vi "retrieveData.vi"(8 "error in (no error)":errorcluster, 11 "DistanceGauge in":refnum<class "DistanceGauge.lvclass">) -> (0 "error out":errorcluster, 2 "Distance Data":T1={"Distance Measured 1"=1.0, "Distance Measured 2"=1.0} {"Distance Measured 2" min=1.0 max=300.0 format="%.1f"; "Distance Measured 1" min=1.0 max=300.0 format="%.1f"}, 3 "DistanceGauge out":refnum<class "DistanceGauge.lvclass">)   [LabVIEW 2013, in "DistanceGauge.lvlib" / "DistanceGauge.lvclass"]
uses:
  <userlib>/Common/Devices/DistanceGauge/DistanceGauge/DistanceGauge.lvclass
  <userlib>/Common/Devices/DistanceGauge/Typedefs/Distance Data.ctl
  <userlib>/Common/Devices/DistanceGauge/DistanceGauge/DistanceGauge.lvclass/DistanceGauge.ctl
  <userlib>/Common/SerialProtocols/SerialCommunicator/SerialCommunicator.lvclass
  <userlib>/Common/Devices/DistanceGauge/DistanceGauge.lvlib
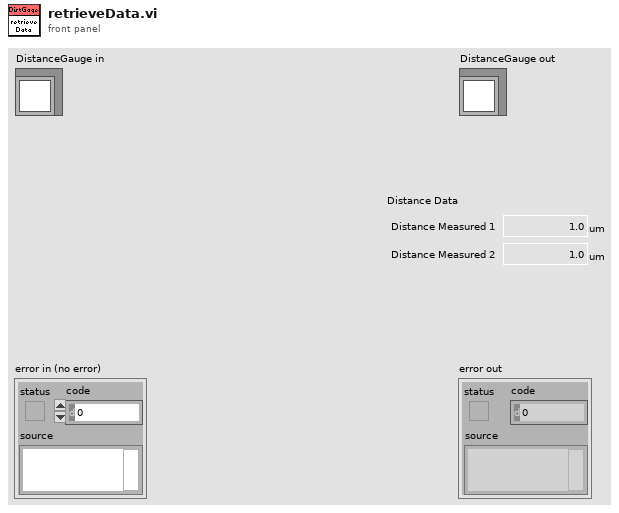
[diagram p1: front panel]
types:
  T1 = typedef "DistanceGauge.lvlib/Distance Data.ctl" = cluster{"Distance Measured 1":dbl[unit], "Distance Measured 2":dbl[unit]}
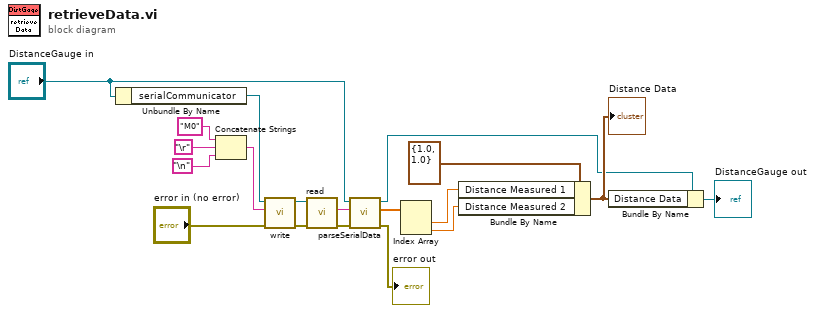
[diagram p0: block diagram]
diagram:
  n1 = Unbundle By Name("DistanceGauge in") -> ("serialCommunicator"=w14:refnum<class "SerialCommunicator.lvclass">)
  n2 = Concatenate Strings("M0" ("writeString"), "\r", "\n") -> (w9:string)
  n3 = call-dynamic "write.vi"("error in (no error)"="error in (no error)", "writeString"=w9, "SerialCommunicator in"=w14) -> ("error out"=w11:errorcluster, "SerialCommunicator out"=w13:refnum<class "SerialCommunicator.lvclass">)  [unwired: 7 in]
  n4 = call-dynamic "read.vi"("error in (no error)"=w11, "SerialCommunicator in"=w13) -> ("error out"=w4:errorcluster, "stringRead"=w2:string)  [unwired: 7 in, 1 out]
  n5 = call <userlib>:"parseSerialData.vi"("error in (no error)"=w4, "serialData"=w2, "DistanceGauge in"="DistanceGauge in") -> ("error out"=→"error out":errorcluster, "dataArray"=w1:dbl[unit][], "DistanceGauge out"=w5:refnum<class "DistanceGauge.lvclass">)  [unwired: 6 in]
  n6 = Index Array(array=w1) -> (element #1=w17:dbl[unit], element #2=w16:dbl[unit])  [unwired: 2 in]
  n7 = Bundle By Name(cluster=T1 {"Distance Measured 1"=1.0, "Distance Measured 2"=1.0} ("Distance Data"), "Distance Measured 1"=w17, "Distance Measured 2"=w16) -> (w15:T1)
  "Distance Data" <- w15
  n8 = Bundle By Name(cluster=w5, "Distance Data"=w15) -> (→"DistanceGauge out":refnum<class "DistanceGauge.lvclass">)
